vi "testMessage.vi"() -> (0 "error out":errorcluster)   [LabVIEW 2017, in "AssertionTest.lvlib" / "AssertEquals.lvlib"]
uses:
  AssertEquals.lvlib
  Assertion/Assertion.lvlib
  10e1fe13-a19d-46b0-b960-6dd61c6be12d.vi
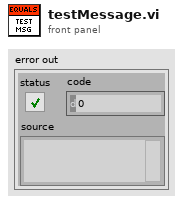
[diagram p1: front panel]
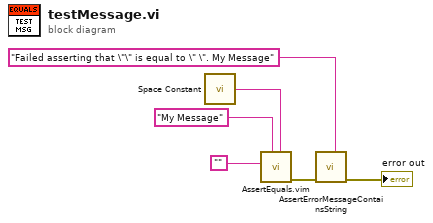
[diagram p0: block diagram]
diagram:
  n1 = call <vilib>:"Space Constant.vi"() -> ("String"=w3:string)
  n2 = call "AssertEquals.vim"("Expected"=w3, "Message (\"\")"="My Message" ("Message (\"\")"), "Actual"="") -> ("error out"=w6:errorcluster)  [unwired: 8 in]
  n3 = call "AssertErrorMessageContainsString.vi"("Expected"="Failed asserting that \"\" is equal to \" \". My Message" ("y"), "error in (no error)"=w6) -> ("error out"=→"error out":errorcluster)  [unwired: 9 in]
